vi "Add.vi"(8 "Add value":dbl, 11 "Score_A":dbl) -> (3 "Score Out":dbl)   [LabVIEW 2021]
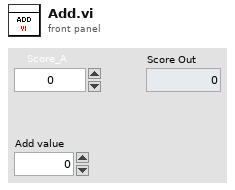
[diagram p1: front panel]
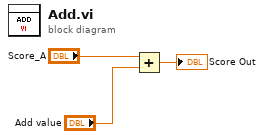
[diagram p0: block diagram]
diagram:
  n1 = Add(x="Score_A", y="Add value") -> (x+y=→"Score Out":dbl)
